vi "Write Name.vi"(10 "Name":string, 11 "Series in":refnum<class "Series.lvclass">) -> (3 "Series out":refnum<class "Series.lvclass">)   [LabVIEW 2018, in "InfluxDB Client.lvlib" / "Series.lvclass"]
uses:
  Series.lvclass
  Series.lvclass/Series.ctl
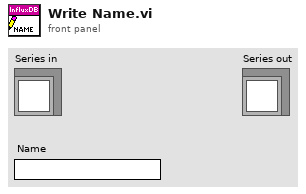
[diagram p1: front panel]
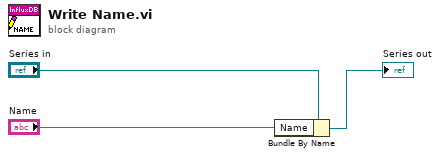
[diagram p0: block diagram]
diagram:
  n1 = Bundle By Name(cluster="Series in", "Name"="Name") -> (→"Series out":refnum<class "Series.lvclass">)
